vi "FFT_DAS_Cont Acq&Graph Voltage-Int Clk.vi"() -> ()   [LabVIEW 2010]
doc: "I. Description:\nThis example demonstrates how to acquire a continuous amount of data (Waveform) using the DAQ device's internal clock.\n\nII. Instructions for Running:\n1. Create an analog input voltage channel.\n2. Set the rate for the sample clock. Additionally, define the sample mode to be continuous.\n3. Call the Start VI to start the acquisition.\n4. Read the waveform data in a loop until the user hits the stop button or an error occurs.\nNote: This example reads data from one or more channels and returns an array of data. Use the Index Array function to access an individual channel of data.\n5. Call the Clear Task VI to clear the Task.\n6. Use the popup dialog box to display an error if any.\n\nIV. I/O Connections Overview:\nMake sure your signal input terminal matches the Physical Channel I/O Control. For further connection information, refer to your hardware reference manual."
uses:
  <vilib>/Utility/error.llb/DialogType.ctl
  <vilib>/DAQmx/read.llb/DAQmx Read (Analog 1D Wfm NChan NSamp).vi
  <vilib>/DAQmx/create/channels.llb/DAQmx Create Channel (AI-Voltage-Basic).vi
  <vilib>/DAQmx/configure/timing.llb/DAQmx Timing (Sample Clock).vi
  <vilib>/daqmx/miscellaneous.llb/DAQmx Fill In Error Info.vi
panel:
  in  "Samples to Read":i32=10
  in  "Physical Channel":tag="Dev1/ai0:3"
  in  "Minimum Value":dbl=-1.0 format="%0.2f"
  in  "Maximum Value":dbl=6.0 format="%0.2f"
  in  "stop":bool
  in  "Sample Rate":dbl=100.0 caption="Sample Rate (Hz)" format="%0.2f"
  out "Measurement":waveform(dbl)[](graph)
  # "For instructions, select Help>>Show Context Help"
  # "Channel Parameters"
  # "Timing Parameters"
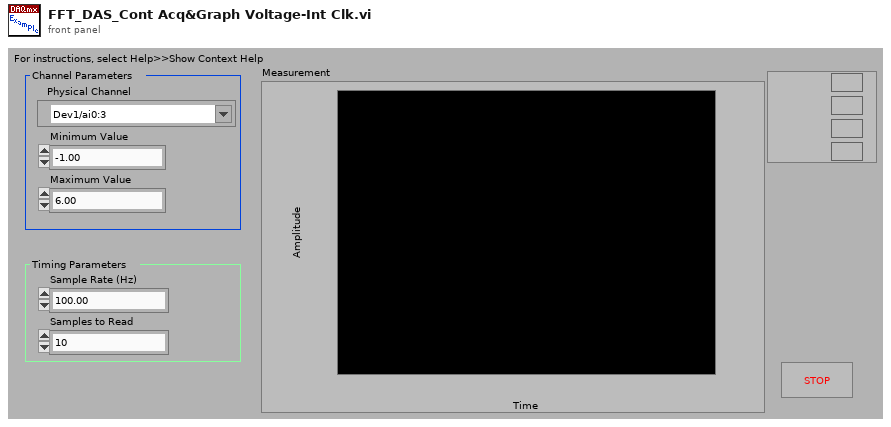
[diagram p1: front panel]
types:
  T1 = typedef "DialogType.ctl" = u16
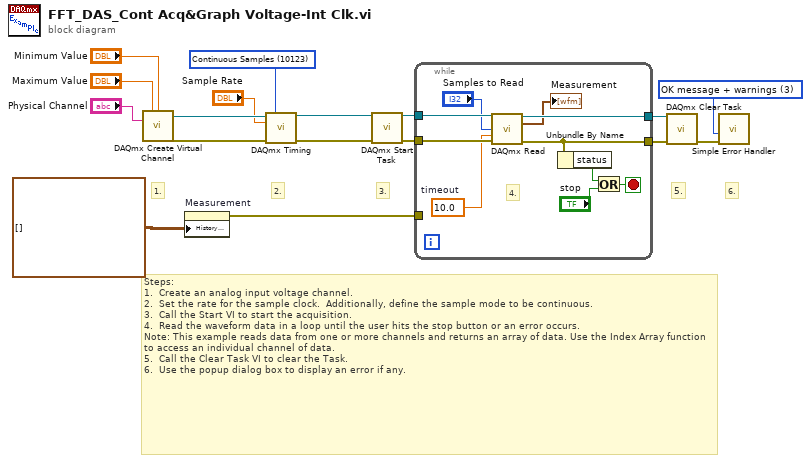
[diagram p0: block diagram]
diagram:
  w3 = T1 3 items=["no dialog", "OK message", "continue or stop message", "OK message + warnings", "continue/stop + warnings"] ("type of dialog (OK msg:1)")
  w8 = 10123 items=["Finite Samples"=10178, "Continuous Samples"=10123] ("sample mode")
  # "6."
  # "5."
  # "Steps: \n1.  Create an analog input voltage channel.\n2.  Set the rate for the sample clock.  Additionally, define the sample mode to be continuous.\n3.  Call the Start VI to start the acquisition.\n4.  Read the waveform data in a loop until the user hits the stop button or an error occurs.\nNote: This example reads data from one or more channels and returns an array of data. Use the Index Array function to access an individual channel of data.\n5.  Call the Clear Task VI to clear the Task.\n6.  Use the popup dialog box to display an error if any."
  # "3."
  # "2."
  # "1."
  n1 = call-poly <vilib>:"DAQmx Create Virtual Channel.vi"("maximum value"="Maximum Value", "minimum value"="Minimum Value", "physical channels"="Physical Channel") -> ("task out"=w12:refnum<k21>, "error out"=w15:errorcluster)  [unwired: 11 in]
  n2 = property on="Measurement" class="WFChart (strict)"("History Data"=waveform(dbl)[][] []) -> (error out=w2:errorcluster)  [unwired: 2 in, 1 out]
  n3 = call-poly <vilib>:"DAQmx Timing.vi"("task/channels in"=w12, "sample mode"=w8, "rate"="Sample Rate", "error in"=w15) -> ("task out"=w7:refnum<k21>, "error out"=w6:errorcluster)  [unwired: 10 in]
  n4 = call <vilib>:"DAQmx Start Task.vi"("task/channels in"=w7, "error in"=w6) -> ("task out"=w11:refnum<k21>, "error out"=w14:errorcluster)  [unwired: 12 in]
  n5 = while {
    tunnel: w14 -> [w27]
    tunnel: w11 -> [w26]
    tunnel: [w25] -> w10
    tunnel: [w23] -> w5
    tunnel: w2 -> [_]
    stop <- w21 stop-if-true
    w19 = 10.0  # timeout
    # "4."
    n6 = call-poly <vilib>:"DAQmx Read.vi"("task/channels in"=w26, "number of samples per channel"="Samples to Read", "timeout"=w19, "error in"=w27) -> ("task out"=w25:refnum<k21>, "data"=→"Measurement":waveform(dbl)[], "error out"=w23:errorcluster)  [unwired: 9 in]
    n7 = Unbundle By Name(w23) -> ("status"=w22:bool)
    n8 = Or(x=w22, y="stop") -> (x .or. y?=w21:bool)
  }
  n9 = call <vilib>:"DAQmx Clear Task.vi"("task in"=w10, "error in"=w5) -> ("error out"=w13:errorcluster)  [unwired: 13 in]
  n10 = call <vilib>:"Simple Error Handler.vi"("type of dialog (OK msg:1)"=w3, "error in (no error)"=w13) -> ()  [unwired: 3 in, 5 out]
